vi "Definition Cluster.vi"(11 "String in":refnum<class "String.lvclass">) -> (2 "Definition":variant, 3 "String out":refnum<class "String.lvclass">)   [LabVIEW 2020, in "Conditu2.lvlib" / "Columns.lvlib" / "String.lvclass"]
uses:
  String.lvclass
  C:/dev/lv20CE/lv-conditum-tools/Conditum-Clone/Columns/Type/Type.lvclass
  String Definition.ctl
  Type/Definition.ctl
  Attributes.ctl
  Definition.ctl
  String.lvclass/String.ctl
  Conditu2.lvlib
  Type/Type.lvclass
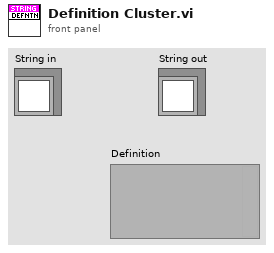
[diagram p1: front panel]
types:
  T1 = typedef "Conditu2.lvlib/Columns.lvlib/String.lvclass/String Definition.ctl" = cluster{"Type":T2, "Attributes":T3, "String":T4}
  T2 = typedef "Conditu2.lvlib/Columns.lvlib/Type.lvclass/Definition.ctl" = cluster{"Name":string, "Nullable":bool, "Default NULL":bool}
  T3 = typedef "Conditu2.lvlib/Attributes.ctl" = cluster{"Primary Key":bool, "Unique":bool, "Foreign Key":bool, "Auto Increment":bool}
  T4 = typedef "Conditu2.lvlib/Columns.lvlib/String.lvclass/Definition.ctl" = cluster{"Default":string, "Length":i32}
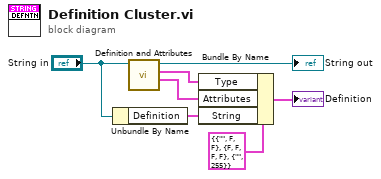
[diagram p0: block diagram]
diagram:
  n1 = Unbundle By Name("String in") -> ("Definition"=w6:T4)
  n2 = call "Definition and Attributes.vi"("Type in"="String in") -> ("Attributes"=w4:T3, "Definition"=w5:T2, "Type out"=→"String out":refnum<class "String.lvclass">)  [unwired: 8 in]
  n3 = Bundle By Name(cluster=T1 {"Type"={"Name"="", "Nullable"=FALSE, "Default NULL"=FALSE}, "Attributes"={"Primary Key"=FALSE, "Unique"=FALSE, "Foreign Key"=FALSE, "Auto Increment"=FALSE}, "String"={"Default"="", "Length"=255}} ("Definition"), "Type"=w5, "Attributes"=w4, "String"=w6) -> (→"Definition":T1)
